vi "LabVIEW_LED_Game.vi"() -> ()   [LabVIEW 2020]
doc: "This VI uses a light pattern game to demonstrate using Event structures to monitor a user's mouse clicks. The VI uses the Mouse Down and Timeout events to determine if the user clicks the correct LED in the appropriate amount of time."
uses:
  simon_colors.ctl
panel:
  out "Current Round":i32
  out "green":bool
  out "yellow":bool
  out "blue":bool
  out "red":bool
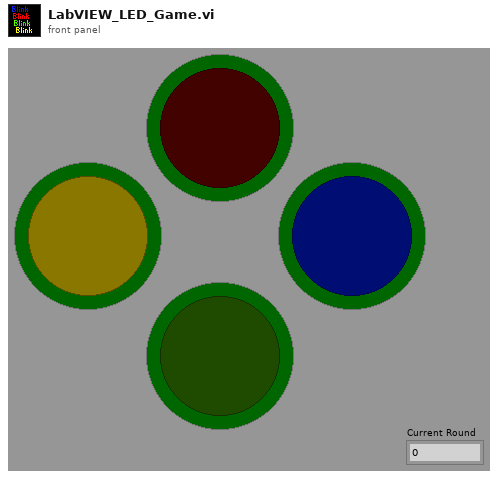
[diagram p1: front panel]
types:
  T1 = typedef "simon_colors.ctl" = enum16{"red", "green", "yellow", "blue"}
  T2 = enum16{"Left Button", "Center Button", "Right Button", "Window Close"}
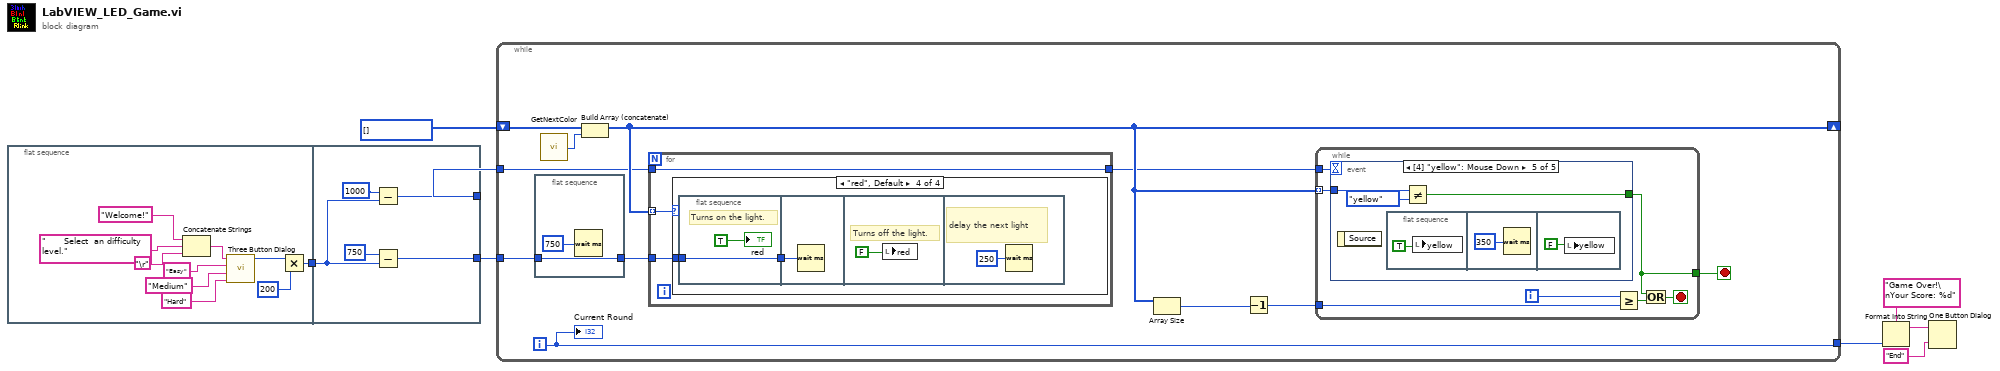
[diagram p0: block diagram]
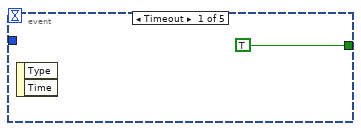
[diagram p2: hidden frame]
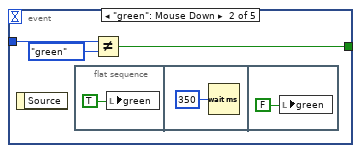
[diagram p3: hidden frame]
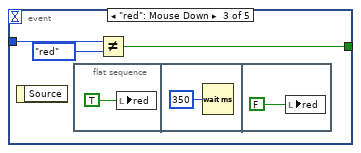
[diagram p4: hidden frame]
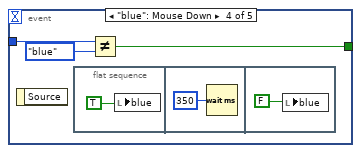
[diagram p5: hidden frame]
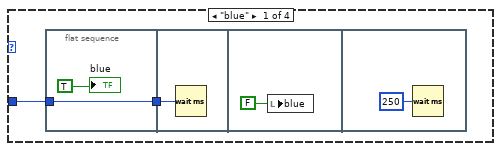
[diagram p6: hidden frame]
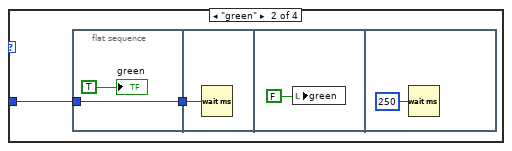
[diagram p7: hidden frame]
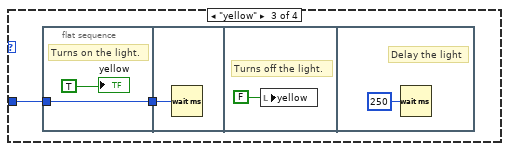
[diagram p8: hidden frame]
diagram:
  w5 = T1[] [] items=["red", "green", "yellow", "blue"]
  n1 = flat-sequence {
    tunnel: [w12] -> w8
    tunnel: w8 -> [w20]
    tunnel: [w22] -> w1
    tunnel: [w19] -> w6
    frame #0 {
      n2 = Concatenate Strings("Welcome!" ("message"), "      Select  an difficulty level." ("string"), "\r") -> (w15:string)
      n3 = call <vilib>:"Three Button Dialog.vi"("Right Button Text (\"Cancel\")"="Hard" ("Right Button Text (\"Cancel\")"), "Center Button Text (\"No\")"="Medium" ("Center Button Text (\"No\")"), "Left Button Text (\"Yes\")"="Easy" ("Left Button Text (\"Yes\")"), "message"=w15) -> ("Which Button?"=w14:T2)  [unwired: 7 in]
      n4 = Multiply(x=w14, y=200) -> (x*y=w12:i32)
    }
    frame #1 {
      n5 = Subtract(x=1000, y=w20) -> (x-y=w22:i32)
      n6 = Subtract(x=u32 750 ("millisecond multiple"), y=w20) -> (x-y=w19:u32)
    }
  }
  n7 = while {
    shift-right: [w31] -> _
    shift-left: w5 -> [w32]
    tunnel: [w34] -> w7
    tunnel: w6 -> [w24]
    tunnel: w1 -> [w27]
    i -> [w34]
    stop <- w28 stop-if-true
    n8 = flat-sequence {
      tunnel: [w36] -> w25
      tunnel: w24 -> [w36]
      frame #0 {
        n9 = Wait (ms)(milliseconds to wait=u32 750 ("millisecond multiple")) -> ()  [unwired: 1 out]
      }
    }
    n10 = call "GetNextColor.vi"() -> ("Color Selected"=w33:T1)  [unwired: 1 in]
    n11 = Build Array (concatenate)(w32, w33) -> (w31:T1[])
    n12 = for {
      tunnel: w31 -> [w71] mode=indexing
      tunnel: w25 -> [w70]
      tunnel: [w69] -> w26
      tunnel: w27 -> [w69]
      n13 = case shown="\"red\", Default" w71 {
        tunnel: w70 -> [w73 w79 w86 w93]
        frame "blue" {
          n14 = flat-sequence {
            tunnel: w73 -> [w75]
            tunnel: [w75] -> w72
            tunnel: w72 -> [w76]
            frame #0 {
              "blue" <- TRUE ("blue")
            }
            frame #1 {
              n15 = Wait (ms)(milliseconds to wait=w76) -> ()  [unwired: 1 out]
            }
            frame #2 {
              n16 = local write "blue"(FALSE ("blue")) -> ()
            }
            frame #3 {
              n17 = Wait (ms)(milliseconds to wait=u32 250 ("millisecond multiple")) -> ()  [unwired: 1 out]
            }
          }
        }
        frame "green" {
          n18 = flat-sequence {
            tunnel: w79 -> [w82]
            tunnel: [w82] -> w80
            tunnel: w80 -> [w83]
            frame #0 {
              "green" <- TRUE ("green")
            }
            frame #1 {
              n19 = Wait (ms)(milliseconds to wait=w83) -> ()  [unwired: 1 out]
            }
            frame #2 {
              n20 = local write "green"(FALSE ("green")) -> ()
            }
            frame #3 {
              n21 = Wait (ms)(milliseconds to wait=u32 250 ("millisecond multiple")) -> ()  [unwired: 1 out]
            }
          }
        }
        frame "yellow" {
          n22 = flat-sequence {
            tunnel: w86 -> [w89]
            tunnel: [w89] -> w87
            tunnel: w87 -> [w90]
            frame #0 {
              # "Turns on the light."
              "yellow" <- TRUE ("yellow")
            }
            frame #1 {
              n23 = Wait (ms)(milliseconds to wait=w90) -> ()  [unwired: 1 out]
            }
            frame #2 {
              # "Turns off the light."
              n24 = local write "yellow"(FALSE ("yellow")) -> ()
            }
            frame #3 {
              # "Delay the light"
              n25 = Wait (ms)(milliseconds to wait=u32 250 ("millisecond multiple")) -> ()  [unwired: 1 out]
            }
          }
        }
        frame "red", Default {
          n26 = flat-sequence {
            tunnel: w93 -> [w96]
            tunnel: [w96] -> w94
            tunnel: w94 -> [w97]
            frame #0 {
              # "Turns on the light."
              "red" <- TRUE ("red")
            }
            frame #1 {
              n27 = Wait (ms)(milliseconds to wait=w97) -> ()  [unwired: 1 out]
            }
            frame #2 {
              # "Turns off the light."
              n28 = local write "red"(FALSE ("red")) -> ()
            }
            frame #3 {
              # "delay the next light"
              n29 = Wait (ms)(milliseconds to wait=u32 250 ("millisecond multiple")) -> ()  [unwired: 1 out]
            }
          }
        }
      }
    }
    n30 = Array Size(array=w31) -> (size(s)=w30:i32)
    n31 = Decrement(x=w30) -> (x-1=w29:i32)
    n32 = while {
      tunnel: w31 -> [w43] mode=indexing
      tunnel: [w41] -> w28
      tunnel: w26 -> [w42]
      tunnel: w29 -> [w39]
      i -> [w40]
      stop <- w37 stop-if-true
      n33 = event shown="[4] \"yellow\": Mouse Down" {
        selector: _ -> [_ _ _ _ _]
        dyn-events: _ -> [_ _ _ _ _]
        timeout: w42 -> [_ _ _ _ _]
        tunnel: w43 -> [_ w46 w52 w58 w65]
        tunnel: [TRUE w45 w51 w57 w63] -> w41
        event Timeout {
          n34 = event-data() -> ()  [unwired: 1 in, 2 out]
        }
        event "green": Mouse Down {
          n35 = event-data() -> ()  [unwired: 1 in, 1 out]
          n36 = flat-sequence {
            frame #0 {
              n37 = local write "green"(TRUE ("red")) -> ()
            }
            frame #1 {
              n38 = Wait (ms)(milliseconds to wait=u32 350) -> ()  [unwired: 1 out]
            }
            frame #2 {
              n39 = local write "green"(FALSE ("red")) -> ()
            }
          }
          n40 = Not Equal?(x=w46, y=simon_colors."green" ("Color Selected")) -> (x != y?=w45:bool)
        }
        event "red": Mouse Down {
          n41 = event-data() -> ()  [unwired: 1 in, 1 out]
          n42 = flat-sequence {
            frame #0 {
              n43 = local write "red"(TRUE ("red")) -> ()
            }
            frame #1 {
              n44 = Wait (ms)(milliseconds to wait=u32 350) -> ()  [unwired: 1 out]
            }
            frame #2 {
              n45 = local write "red"(FALSE ("red")) -> ()
            }
          }
          n46 = Not Equal?(x=w52, y=simon_colors."red" ("Color Selected")) -> (x != y?=w51:bool)
        }
        event "blue": Mouse Down {
          n47 = event-data() -> ()  [unwired: 1 in, 1 out]
          n48 = flat-sequence {
            frame #0 {
              n49 = local write "blue"(TRUE ("red")) -> ()
            }
            frame #1 {
              n50 = Wait (ms)(milliseconds to wait=u32 350) -> ()  [unwired: 1 out]
            }
            frame #2 {
              n51 = local write "blue"(FALSE ("red")) -> ()
            }
          }
          n52 = Not Equal?(x=w58, y=simon_colors."blue" ("Color Selected")) -> (x != y?=w57:bool)
        }
        event "yellow": Mouse Down {
          n53 = event-data() -> ()  [unwired: 1 in, 1 out]
          n54 = flat-sequence {
            frame #0 {
              n55 = local write "yellow"(TRUE ("red")) -> ()
            }
            frame #1 {
              n56 = Wait (ms)(milliseconds to wait=u32 350) -> ()  [unwired: 1 out]
            }
            frame #2 {
              n57 = local write "yellow"(FALSE ("red")) -> ()
            }
          }
          n58 = Not Equal?(x=w65, y=simon_colors."yellow" ("Color Selected")) -> (x != y?=w63:bool)
        }
      }
      n59 = Greater Or Equal?(x=w40, y=w39) -> (x >= y?=w38:bool)
      n60 = Or(x=w41, y=w38) -> (x .or. y?=w37:bool)
    }
    "Current Round" <- w34
  }
  n61 = Format Into String(format string="Game Over!\nYour Score: %d" ("initial string"), w7) -> (resulting string=w2:string)  [unwired: 2 in, 1 out]
  n62 = One Button Dialog(message=w2, button name ("OK")="End") -> ()  [unwired: 1 out]
